vi "CreatePrivateEvents.vi"(8 "error in (no error)":errorcluster, 11 "XYStage.KIM101":refnum<class "XYStage.KIM101.lvclass">) -> (0 "error out":errorcluster, 3 "XYStage.KIM101 out":refnum<class "XYStage.KIM101.lvclass">)   [LabVIEW 2019, in "XYStage.KIM101.lvclass"]
doc: "JKI State Machine Objects (SMO) 1.3.0.56\nJKI - JKI\nCopyright (c) 2017, JKI"
uses:
  XYStage.KIM101.lvclass
  XYStage.KIM101.lvclass/XYStage.KIM101.ctl
  Typedefs/PrivateEvents--XYStage.KIM101.MoveAbsolute (counts).ctl
  XYStage/Typedefs/Coordinates.Counts--Cluster.ctl
  XYStage/XYStage.lvclass
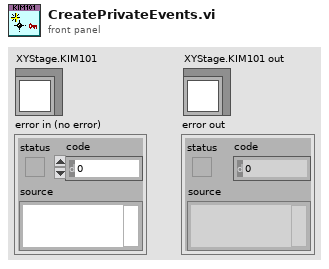
[diagram p1: front panel]
types:
  T1 = typedef "XYStage.KIM101.lvclass/PrivateData--Ref.ctl" = refnum<data-value>
  T2 = typedef "XYStage.KIM101.lvclass/PrivateEvents--XYStage.KIM101.MoveAbsolute (counts).ctl" = cluster{"Coordinates.Counts":T3, "Wait Timeout, ms":i32}
  T3 = typedef "XYStage.lvclass/Coordinates.Counts--Cluster.ctl" = cluster{"X":i32, "Y":i32}
  T4 = typedef "XYStage.KIM101.lvclass/PrivateData--Cluster.ctl" = cluster{"Resource":T5, "Private Events":T6}
  T5 = typedef "XYStage.KIM101.lvclass/Resource--Cluster.ctl" = cluster{"KCubeInertialMotorControl":refnum<k24>, "Device":refnum<k24>, "X Axis Channel":i32, "Y Axis Channel":i32}
  T6 = typedef "XYStage.KIM101.lvclass/PrivateEvents--Cluster.ctl" = cluster{"MoveAbsolute (counts)":refnum<user-event>}
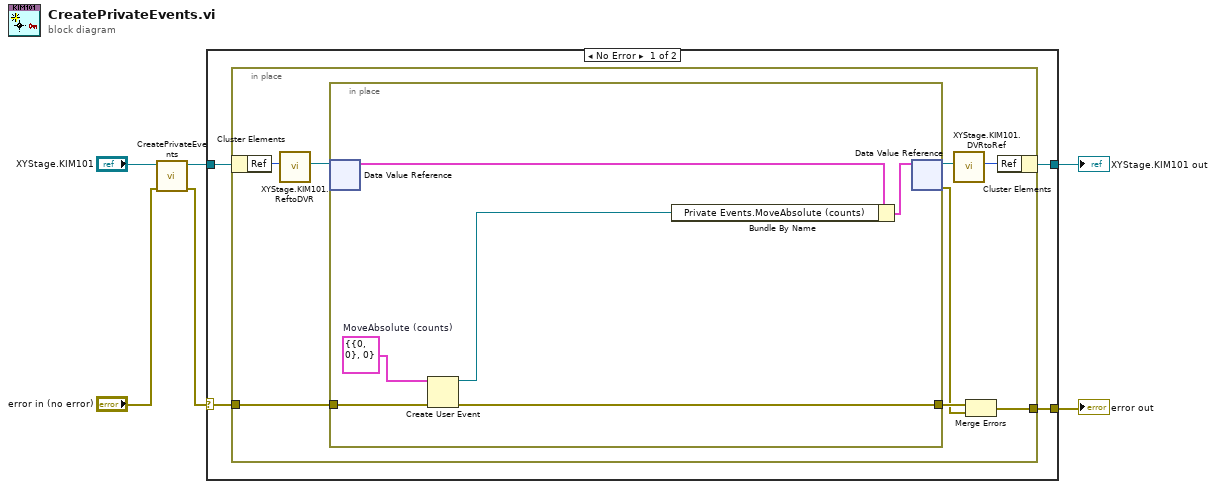
[diagram p0: block diagram]
diagram:
  n1 = call-parent "CreatePrivateEvents.vi"("error in (no error)"="error in (no error)", "XYStage"="XYStage.KIM101") -> ("error out"=w4:errorcluster, "XYStage out"=w3:refnum<class "XYStage.KIM101.lvclass">)  [unwired: 8 in]
  n2 = case shown="No Error" w4 {
    selector: w4 -> [w9 w26]
    tunnel: w3 -> [w10 w25]
    tunnel: [w8 w26] -> w2
    tunnel: [w7 w25] -> w1
    frame No Error {
      n3 = in-place {
        in-place-border: w9 -> [w15]
        in-place-border: [w12] -> w8
        n4 = in-place-cluster #1(w10) -> ("Ref"=w18:u32)
        n5 = call "XYStage.KIM101.ReftoDVR.vi"("Ref"=w18) -> ("Ref"=w16:T1)  [unwired: 10 in]
        n6 = in-place {
          in-place-border: w15 -> [w22]
          in-place-border: [w21] -> w14
          w20 = T2 {"Coordinates.Counts"={"X"=0, "Y"=0}, "Wait Timeout, ms"=0}  # MoveAbsolute (counts)
          n7 = in-place-dvr #2(w16) -> (w24:T4)  [unwired: 1 out]
          n8 = Create User Event(user event datatype=w20, error in=w22) -> (user event=w19:refnum<user-event>, error out=w21:errorcluster)
          n9 = Bundle By Name(cluster=w24, "Private Events.MoveAbsolute (counts)"=w19) -> (w23:T4)
          n10 = in-place-dvr #2(w23) -> (w11:T1, w13:errorcluster)
        }
        n11 = call "XYStage.KIM101.DVRtoRef.vi"("Ref"=w11) -> ("Ref"=w17:u32)  [unwired: 10 in]
        n12 = Merge Errors(w14, w13) -> (w12:errorcluster)
        n13 = in-place-cluster #1("Ref"=w17) -> (w7:refnum<class "XYStage.KIM101.lvclass">)
      }
    }
    frame Error {
    }
  }
  "error out" <- w2
  "XYStage.KIM101 out" <- w1
